vi "TI Sensored BLDC (FPGA).vi"() -> ()   [LabVIEW 2013]
uses:
  <vilib>/Platform/TimedLoop/XDataNode/timing_clust.ctl
  <vilib>/Platform/TimedLoop/XDataNode/nitl_modes.ctl
  <vilib>/Platform/TimedLoop/XDataNode/wakeup.ctl
  <vilib>/rvi/Emulation/niFpgaSctlEmulationGetInTimedLoop.vi
  <vilib>/rvi/Emulation/niFpgaEmulationReportErrorSimple.vi
  <vilib>/rvi/Emulation/niFpgaGetClockAttributes.vi
  <vilib>/rvi/Emulation/niFpgaCriticalErrorInLSC.vi
  <vilib>/rvi/eio/common/nirviEmuTemplateMethod_errors.vi
  <vilib>/Platform/TimedLoop/XDataNode/XDataNode.xnode
  <vilib>/eio/EIONode/EIONode.xnode
  <vilib>/Platform/TimedLoop/XDataNode/XDNodeRunTimeDep.lvlib
  <vilib>/rvi/Arithmetic/AddSubMult/XNode/nirviSatArithmetic.xnode
panel:
  out "Telapsed (Ticks)":u32
  out "PWM Clock":bool=TRUE
  out "PWM DO":bool
  out "Changed?":bool
  in  "PWM Duty Cycle (Ticks)":i32=1000
  in  "PWM Period (Ticks)":u32=4000
  in  "Min Period (Ticks)":u32=1000
  out "Current Phase":u8=32
  in  "Manual Phase":u8=1
  in  "Manual":bool=TRUE
  in  "Align":bool
  in  "PWM Enable":bool=TRUE
  in  "Phase Positions":i32[](array[numeric])=[0, 120, 240, 360, 480, 600, 720, 840, 960, 1080, 1200, 1320, 1440]
  out "AI Data":fxp<+/-,64,44>[](array[numeric])=[0.21224212646484375, 0.3561267852783203, 0.3583641052246094, 0.35996246337890625]
  in  "AI Loop (uSec)":u32
  out "AI Loop Actual":u32=20
  in  "Position Reset":bool
  in  "Velocity Interval (uSec)":u32=1000
  out "Position (Counts)":i32=589
  out "Acceleration":i32
  out "Velocity":i32
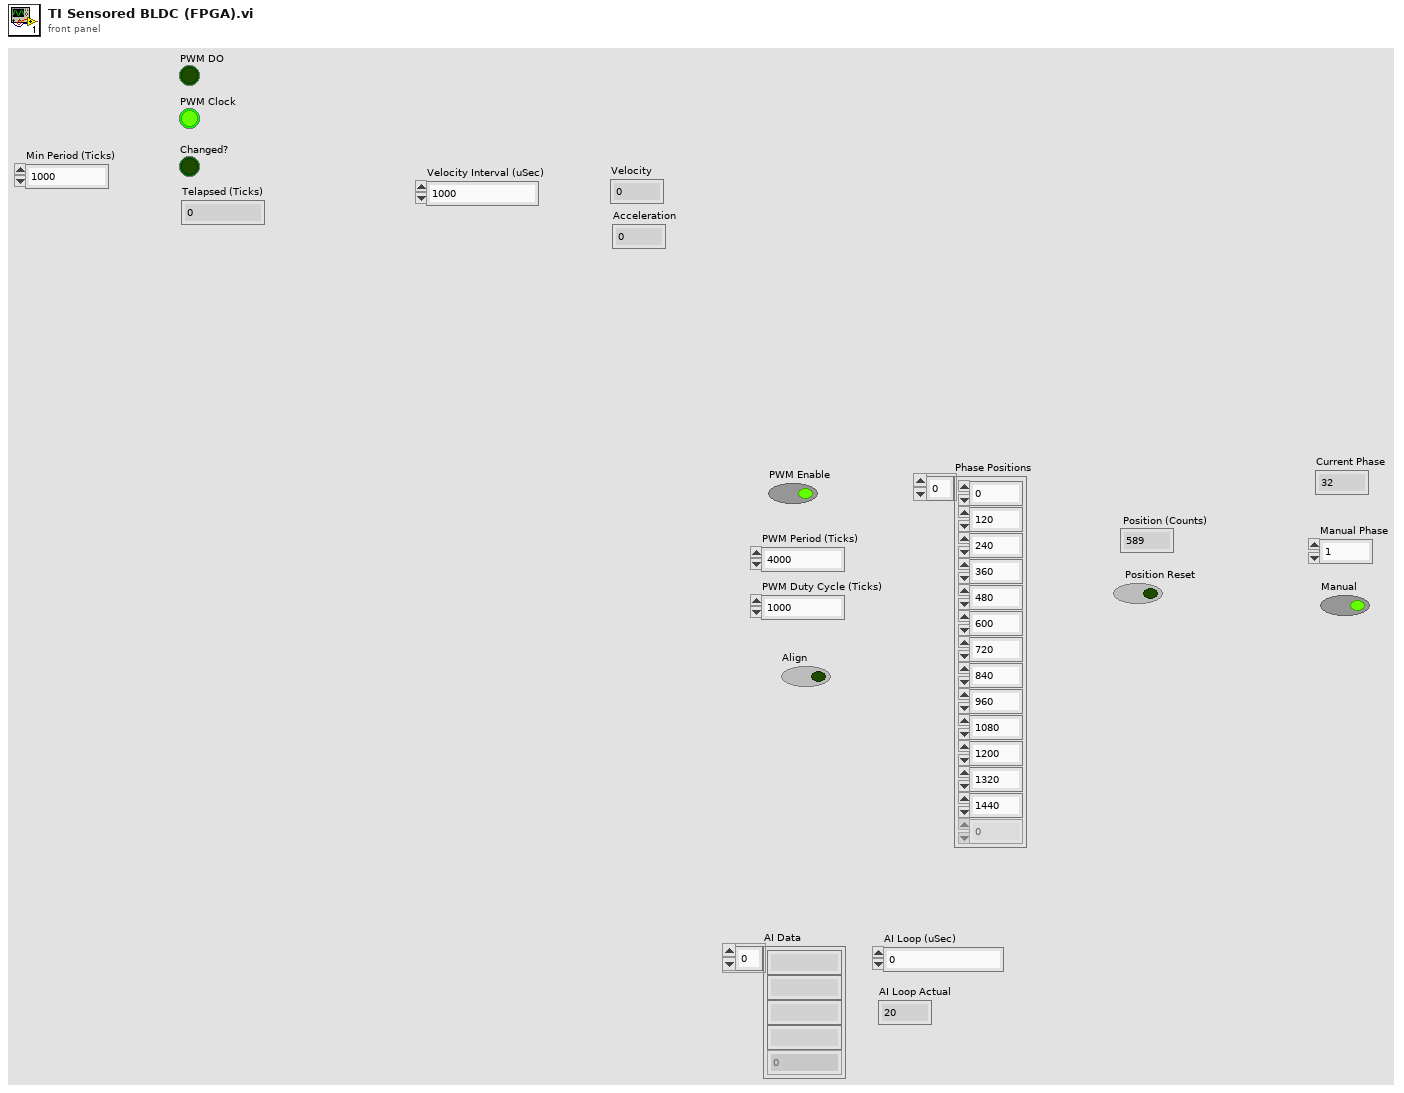
[diagram p1: front panel]
types:
  T1 = typedef "XDNodeRunTimeDep.lvlib/timing_clust.ctl" = cluster{"Expected End [f-1]":u64, "Actual End [f-1]":u64, "Finished Late? [f-1]":bool, "Expected End [i-1]":u64, "Actual End [i-1]":u64, "Finished Late? [i-1]":bool, "Expected Start [i]":u64, "Actual Start [i]":u64, "Expected Start [f]":u64, "Actual Start [f]":u64, "Source Name":string, "Structure Name":string, "Period":i64, "Deadline":i64, "Offset":i64, "Start":i64, "Priority":i32, "Timeout":i32, "Mode":T2, "Wakeup Reason":T3, "Error":errorcluster, "Source Type":string, "Secondary Source Type":string, "Global End Time":u64, "Global Start Time":u64, "Frame Duration":u64, "Iteration Duration":u64, "Assigned CPU":i32, "I/O Scan Engine Mode":u32}
  T2 = typedef "XDNodeRunTimeDep.lvlib/nitl_modes.ctl" = enum32{"No Change", "Process missed periods, maintain original phase", "Discard missed periods, maintain original phase", "Process missed periods, ignore original phase", "Discard missed periods, ignore original phase"}
  T3 = typedef "XDNodeRunTimeDep.lvlib/wakeup.ctl" = enum32{"Normal", "Aborted", "Asynchronous wakeup", "Timing source error", "Timed loop error", "Timeout"}
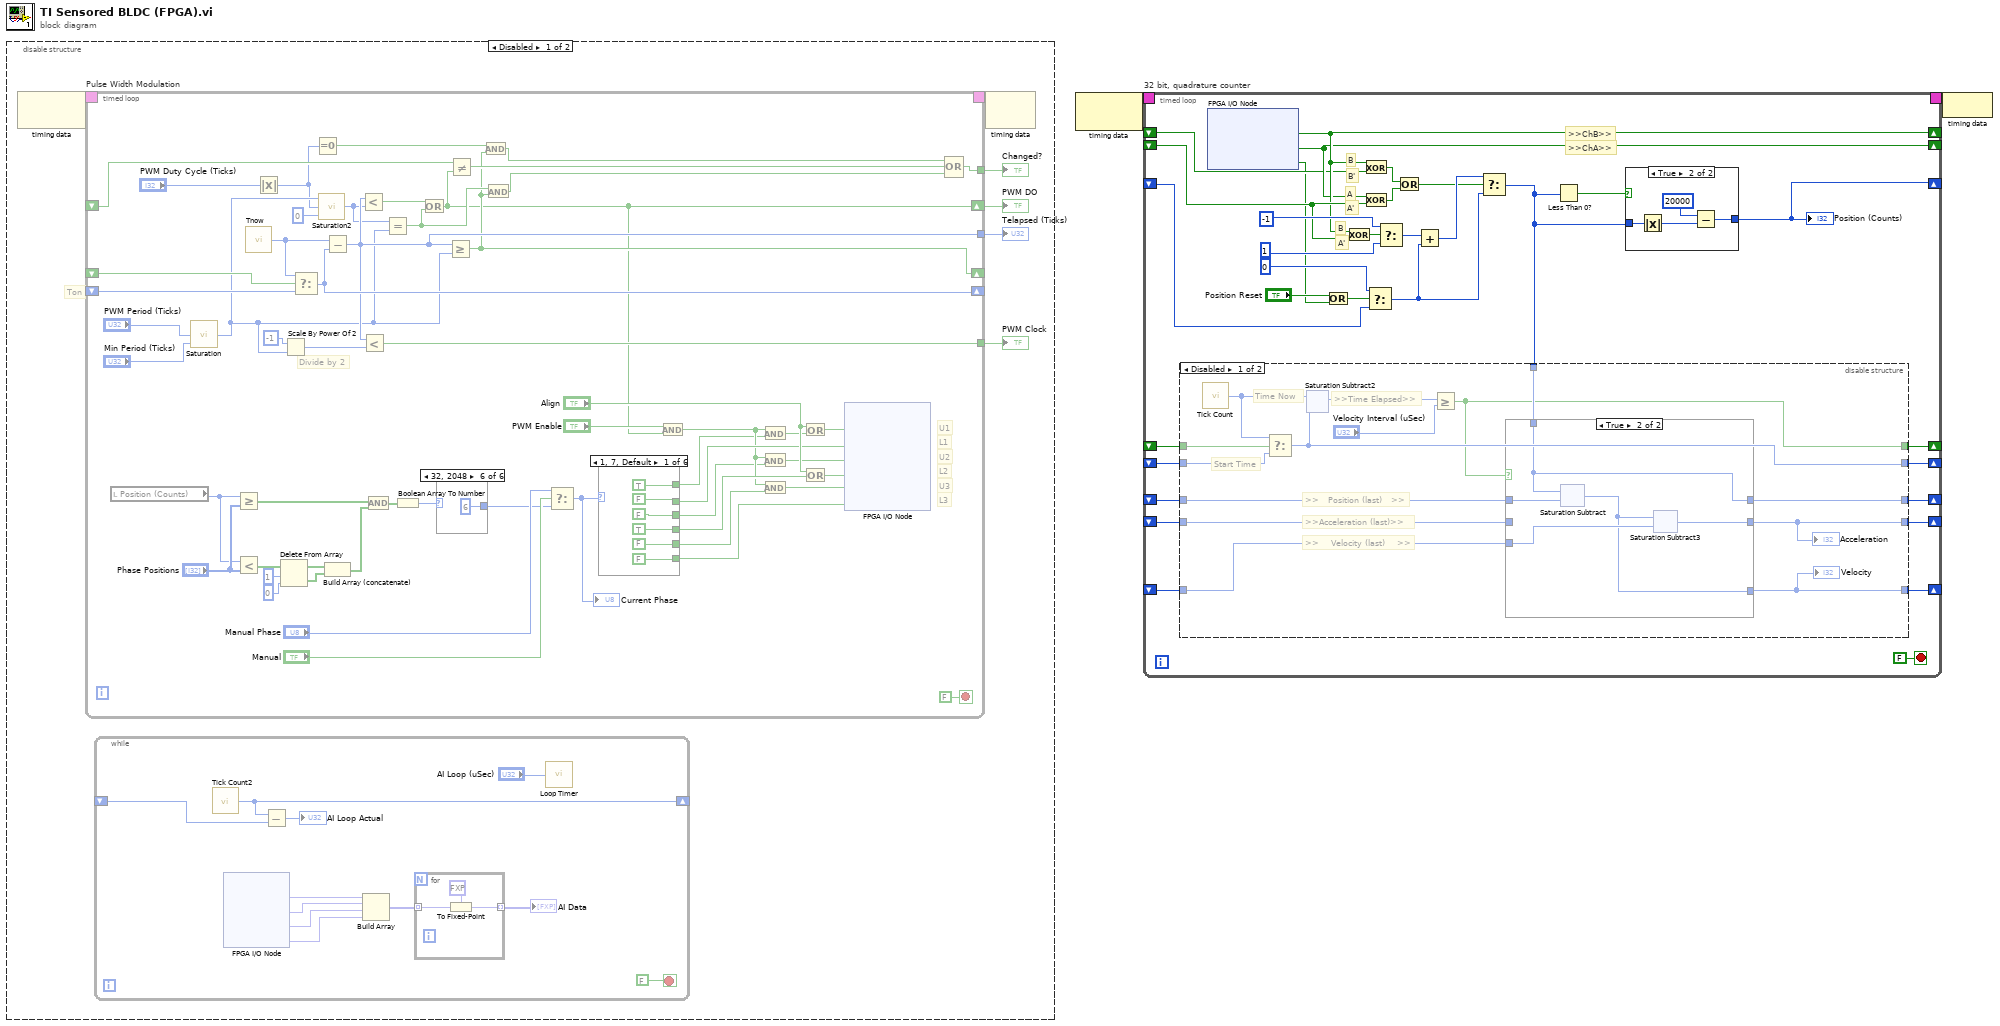
[diagram p0: block diagram]
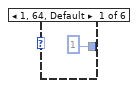
[diagram p2: hidden frame]
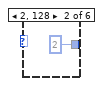
[diagram p3: hidden frame]
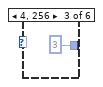
[diagram p4: hidden frame]
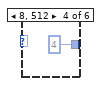
[diagram p5: hidden frame]
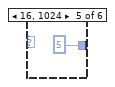
[diagram p6: hidden frame]
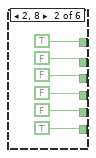
[diagram p7: hidden frame]
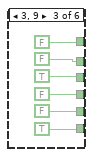
[diagram p8: hidden frame]
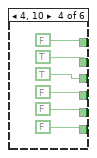
[diagram p9: hidden frame]
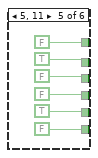
[diagram p10: hidden frame]
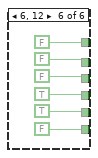
[diagram p11: hidden frame]
diagram:
  n1 = disable-structure shown="Disabled" {
    frame Disabled {
      # "Ton"
      n2 = node-c288() -> (w8:T1)  [unwired: 1 in]
      n3 = timed-loop "Pulse Width Modulation" {
        shift-right: [w59] -> _
        shift-left: _ -> [w60]
        shift-right: [w41] -> _
        shift-left: _ -> [w62]
        tunnel: [w56] -> w3
        tunnel: [w55] -> w4
        shift-right: [w12] -> w5
        shift-left: _ -> [w54]
        tunnel: [w45] -> w6
        timing: w8 -> [_]
        timing-out: [_] -> w7
        stop <- FALSE stop-if-true
        # "L3"
        # "U3"
        # "L2"
        # "U2"
        # "L1"
        # "U1"
        # "Divide by 2"
        n4 = local read "Position (Counts)"() -> (w28:i32)
        n5 = call "Saturation"("input"="PWM Period (Ticks)", "lower limit"="Min Period (Ticks)") -> ("output"=w50:u32)  [unwired: 7 in]
        n6 = Greater Or Equal?(x=w28, y="Phase Positions") -> (x >= y?=w37:bool[])
        n7 = Less?(x=w28, y="Phase Positions") -> (x < y?=w32:bool[])
        n8 = call "Tnow"() -> ("Tick Count(Ticks)"=w61:u32)
        n9 = Absolute Value(x="PWM Duty Cycle (Ticks)") -> (abs(x)=w40:i32)
        n10 = Delete From Array(array=w32, length=1, index=0) -> (deleted portion=w36:bool[], array with subset deleted=w35:bool[])
        n11 = Scale By Power Of 2(n=i8 -1, x=w50) -> (x*2^n=w58:u32)
        n12 = Select(t=w61, s=w62, f=w60) -> (s? t:f=w59:u32)
        n13 = Equal To 0?(x=w40) -> (x = 0?=w39:bool)
        n14 = call "Saturation2"("upper limit"=w50, "input"=w40, "lower limit"=u32 0) -> ("output"=w51:u32)  [unwired: 6 in]
        n15 = Subtract(x=w61, y=w59) -> (x-y=w56:u32)
        n16 = Build Array (concatenate)(w35, w36) -> (w38:bool[])
        n17 = Less?(x=w56, y=w51) -> (x < y?=w49:bool)
        n18 = Less?(x=w56, y=w58) -> (x < y?=w55:bool)
        n19 = And(x=w37, y=w38) -> (x .and. y?=w27:bool[])
        n20 = Equal?(x=w51, y=w50) -> (x = y?=w43:bool)
        n21 = Boolean Array To Number(Boolean array=w27) -> (number=w11:u16)
        n22 = Or(x=w49, y=w43) -> (x .or. y?=w12:bool)
        n23 = case shown="32, 2048" w11 {
          tunnel: [u8 1 ("Manual Phase") u8 2 ("Manual Phase") u8 3 ("Manual Phase") u8 4 ("Manual Phase") u8 5 ("Manual Phase") u8 6 ("Manual Phase")] -> w10
          frame 1, 64, Default {
          }
          frame 2, 128 {
          }
          frame 4, 256 {
          }
          frame 8, 512 {
          }
          frame 16, 1024 {
          }
          frame 32, 2048 {
          }
        }
        n24 = Greater Or Equal?(x=w56, y=w50) -> (x >= y?=w41:bool)
        n25 = Not Equal?(x=w54, y=w12) -> (x != y?=w53:bool)
        n26 = And(x=w39, y=w41) -> (x .and. y?=w42:bool)
        n27 = And(x=w43, y=w41) -> (x .and. y?=w44:bool)
        n28 = Select(t="Manual Phase", s="Manual", f=w10) -> (s? t:f=w9:u8)
        "Current Phase" <- w9
        n29 = case shown="1, 7, Default" w9 {
          tunnel: [FALSE TRUE TRUE FALSE FALSE FALSE] -> w20
          tunnel: [FALSE FALSE FALSE FALSE TRUE TRUE] -> w16
          tunnel: [TRUE FALSE FALSE FALSE FALSE TRUE] -> w26
          tunnel: [FALSE FALSE TRUE TRUE FALSE FALSE] -> w15
          tunnel: [FALSE FALSE FALSE TRUE TRUE FALSE] -> w21
          tunnel: [TRUE TRUE FALSE FALSE FALSE FALSE] -> w14
          frame 1, 7, Default {
          }
          frame 2, 8 {
          }
          frame 3, 9 {
          }
          frame 4, 10 {
          }
          frame 5, 11 {
          }
          frame 6, 12 {
          }
        }
        n30 = And(x="PWM Enable", y=w12) -> (x .and. y?=w19:bool)
        n31 = And(x=w19, y=w14) -> (x .and. y?=w22:bool)
        n32 = And(x=w19, y=w15) -> (x .and. y?=w17:bool)
        n33 = And(x=w19, y=w16) -> (x .and. y?=w18:bool)
        n34 = Or(x="Align", y=w22) -> (x .or. y?=w23:bool)
        n35 = Or(x="Align", y=w26) -> (x .or. y?=w24:bool)
        n36 = xnode "FPGA I/O Node"("RMC/DIO0"=w23, "RMC/DIO1"=w21, "RMC/DIO2"=w17, "RMC/DIO3"=w24, "RMC/DIO4"=w18, "RMC/DIO5"=w20) -> ()  [unwired: 7 in, 7 out]
        n37 = Compound Arithmetic op=OR(w42, w53, w44) -> (w45:bool)
      }
      "Telapsed (Ticks)" <- w3
      "PWM Clock" <- w4
      "PWM DO" <- w5
      "Changed?" <- w6
      n38 = while {
        shift-right: [w117] -> _
        shift-left: _ -> [w116]
        stop <- FALSE stop-if-true
        n39 = call "Tick Count2"() -> ("Tick Count(uSec)"=w117:u32)
        n40 = xnode "FPGA I/O Node"() -> ("AI0"=w111:fxp<+/-,24,5>, "AI1"=w114:fxp<+/-,24,5>, "AI2"=w113:fxp<+/-,24,5>, "AI3"=w112:fxp<+/-,24,5>)  [unwired: 4 in, 4 out]
        n41 = Subtract(x=w117, y=w116) -> (x-y=→"AI Loop Actual":u32)
        n42 = Build Array(w111, w114, w113, w112) -> (w119:fxp<+/-,24,5>[])
        n43 = for {
          tunnel: w119 -> [w123] mode=indexing
          tunnel: [w121] -> w110 mode=indexing
          n44 = To Fixed-Point(fixed-point type=fxp<+/-,64,44> 0.0 ("AI0"), number=w123) -> (fixed-point=w121:fxp<+/-,64,44>)
        }
        "AI Data" <- w110
        n45 = call "Loop Timer"("Count(uSec)"="AI Loop (uSec)") -> ()  [unwired: 1 out]
      }
      n46 = node-c288(w7) -> ()  [unwired: 1 out]
    }
    frame Enabled {
    }
  }
  n47 = node-c288() -> (w2:T1)  [unwired: 1 in]
  n48 = timed-loop "32 bit, quadrature counter" {
    shift-right: [w145] -> _
    shift-left: _ -> [w135]
    shift-right: [w127] -> _
    shift-left: _ -> [w130]
    shift-right: [w144] -> _
    shift-left: _ -> [w146]
    shift-right: [w133] -> _
    shift-left: _ -> [w141]
    shift-right: [w137] -> _
    shift-left: _ -> [w140]
    shift-right: [w134] -> _
    shift-left: _ -> [w139]
    shift-right: [w131] -> _
    shift-left: _ -> [w138]
    shift-right: [w132] -> _
    shift-left: _ -> [w136]
    timing: w2 -> [_]
    timing-out: [_] -> w1
    stop <- FALSE ("stop") stop-if-true
    # "A'"
    # "B"
    # "A'"
    # "A"
    # "B'"
    # "B"
    # ">>ChB>>"
    # ">>ChA>>"
    n49 = xnode "FPGA I/O Node"() -> ("RMC/DIO49"=w145:bool, "RMC/DIO48"=w144:bool, "RMC/DIO50"=w125:bool)  [unwired: 3 in, 3 out]
    n50 = Or(x="Position Reset", y=w125) -> (x .or. y?=w124:bool)
    n51 = Exclusive Or(1:w146, 2:w145) -> (0:w147:bool)
    n52 = Exclusive Or(1:w135, 2:w145) -> (0:w148:bool)
    n53 = Exclusive Or(1:w146, 2:w144) -> (0:w149:bool)
    n54 = Select(t=0 ("32 bit"), s=w124, f=w130) -> (s? t:f=w153:i32)
    n55 = Select(t=-1 ("32 bit"), s=w147, f=1 ("32 bit")) -> (s? t:f=w152:i32)
    n56 = Or(x=w148, y=w149) -> (x .or. y?=w142:bool)
    n57 = Add(x=w152, y=w153) -> (x+y=w155:i32)
    n58 = Select(t=w155, s=w142, f=w153) -> (s? t:f=w128:i32)
    n59 = disable-structure shown="Disabled" {
      disable-tunnel: w141 -> [w174 _]
      disable-tunnel: w140 -> [w173 _]
      disable-tunnel: w139 -> [w171 _]
      disable-tunnel: w138 -> [w170 _]
      disable-tunnel: [w168 _] -> w137
      disable-tunnel: w136 -> [w167 _]
      disable-tunnel: [w166 _] -> w134
      disable-tunnel: w128 -> [w164 _]
      disable-tunnel: [w163 _] -> w133
      disable-tunnel: [w162 _] -> w132
      disable-tunnel: [w161 _] -> w131
      frame Disabled {
        # ">>Acceleration (last)>>"
        # "Start Time"
        # ">>    Velocity (last)    >>"
        # ">>   Position (last)   >>"
        # "Time Now"
        # ">>Time Elapsed>>"
        n60 = call "Tick Count"() -> ("Tick Count(uSec)"=w169:u32)
        n61 = Select(t=w169, s=w174, f=w173) -> (s? t:f=w168:u32)
        n62 = xnode ("Saturation Subtract2")("x"=w169, "y"=w168) -> ("x-y"=w172:u32)
        n63 = Greater Or Equal?(x=w172, y="Velocity Interval (uSec)") -> (x >= y?=w163:bool)
        n64 = case shown="True" w163 {
          tunnel: w164 -> [_ w190]
          tunnel: w171 -> [w185 w192]
          tunnel: [w187 w189] -> w161
          tunnel: w170 -> [w187 w191]
          tunnel: [w186 w188] -> w162
          tunnel: w167 -> [w186 _]
          tunnel: [w185 w190] -> w166
          frame False {
          }
          frame True {
            n65 = xnode ("Saturation Subtract")("x"=w190, "y"=w192) -> ("x-y"=w189:i32)
            n66 = xnode ("Saturation Subtract3")("x"=w189, "y"=w191) -> ("x-y"=w188:i32)
          }
        }
        "Acceleration" <- w162
        "Velocity" <- w161
      }
      frame Enabled {
      }
    }
    n67 = Less Than 0?(x=w128) -> (x < 0?=w129:bool)
    n68 = case shown="True" w129 {
      tunnel: w128 -> [w156 w160]
      tunnel: [w156 w157] -> w127
      frame False {
      }
      frame True {
        n69 = Absolute Value(x=w160) -> (abs(x)=w159:i32)
        n70 = Subtract(x=20000, y=w159) -> (x-y=w157:i32)
      }
    }
    "Position (Counts)" <- w127
  }
  n71 = node-c288(w1) -> ()
